vi "AWGN.vi"(10 "SNR (dB)":dbl, 11 "Dynamic Data":dynamicdata(waveform)) -> (3 "DC with Gaussian Noise":dynamicdata(waveform))   [LabVIEW 2013]
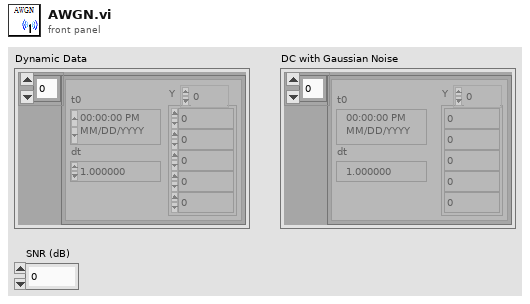
[diagram p1: front panel]
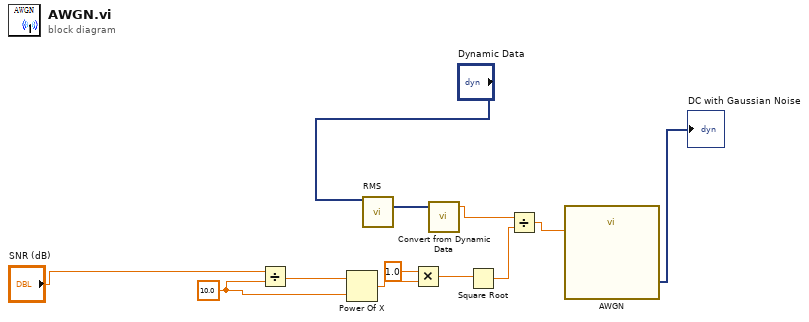
[diagram p0: block diagram]
diagram:
  w7 = 10.0 ("y")
  n1 = Divide(x="SNR (dB)", y=w7) -> (x/y=w8:dbl)
  n2 = Power Of X(1:w7, 2:w8) -> (0:w9:dbl)
  n3 = call "RMS"("Signals"="Dynamic Data") -> ("RMS"=w3:dynamicdata)  [unwired: 13 in, 1 out]
  n4 = Multiply(x=1.0, y=w9) -> (x*y=w11:dbl)
  n5 = call "Convert from Dynamic Data"("Dynamic Data Type"=w3) -> ("Scalar"=w4:dbl)  [unwired: 3 in]
  n6 = Square Root(x=w11) -> (sqrt(x)=w12:dbl)
  n7 = Divide(x=w4, y=w12) -> (x/y=w5:dbl)
  n8 = call "AWGN"("Standard deviation"=w5) -> ("DC with Gaussian Noise"=→"DC with Gaussian Noise":dynamicdata)  [unwired: 13 in, 1 out]
